vi "XY Graph Save Plot Event.vi"(6 "Delimiter (TAB)":string="\t", 8 "Error In":errorcluster, 9 "Mouse Click Coordinates":T1, 11 "XYGraph Ref":T2) -> (0 "Error Out":errorcluster, 1 "Message":string, 2 "File Path":path, 3 "Plot Name":string, 4 "Saved Plot Index":i32, 5 "Graph Caption":string)   [LabVIEW 2019, in "XY Graph Add-Ons.lvlib"]
uses:
  XY Graph Add-Ons.lvlib
  XY Graph Refnum.ctl
  <vilib>/Utility/miscctls.llb/LVPoint32TypeDef.ctl
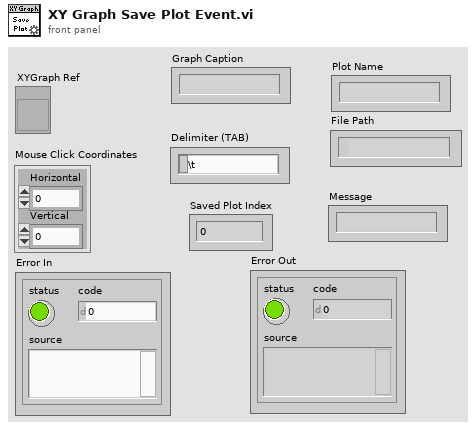
[diagram p1: front panel]
types:
  T1 = typedef "LVPoint32TypeDef.ctl" = cluster{"Horizontal":i32, "Vertical":i32}
  T2 = typedef "XY Graph Add-Ons.lvlib/XY Graph Refnum.ctl" = refnum<vi>
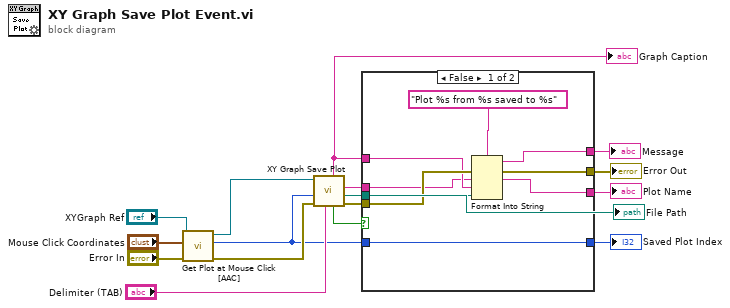
[diagram p0: block diagram]
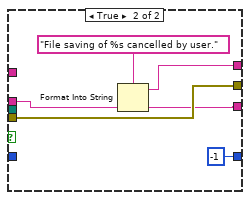
[diagram p2: hidden frame]
diagram:
  n1 = call "Get Plot at Mouse Click [AAC].vi"("error in (no error)"="Error In", "Mouse Click Coordinates"="Mouse Click Coordinates", "XYGraph Ref"="XYGraph Ref") -> ("error out"=w12:errorcluster, "Plot at Coordinates"=w3:i32, "XYGraph Ref"=w14:T2)  [unwired: 2 in, 4 out]
  n2 = call "XY Graph Save Plot.vi"("Delimiter (TAB)"="Delimiter (TAB)", "Error In"=w12, "Plot Index"=w3, "XYGraph Ref"=w14) -> ("Error Out"=w10:errorcluster, "File Path"=w9:path, "Plot Name"=w5:string, "Cancelled"=w4:bool, "Graph Name"=w6:string)  [unwired: 2 in, 1 out]
  "Graph Caption" <- w6
  "File Path" <- w9
  n3 = case shown="False" w4 {
    tunnel: w10 -> [w23 w29]
    tunnel: w9 -> [w22 _]
    tunnel: [w21 w29] -> w8
    tunnel: [w20 w25] -> w7
    tunnel: w6 -> [w19 _]
    tunnel: w5 -> [w17 w26]
    tunnel: w3 -> [w18 _]
    tunnel: [w18 -1 ("Plot at Coordinates")] -> w2
    tunnel: [w17 w26] -> w1
    frame False {
      n4 = Format Into String(format string="Plot %s from %s saved to %s", error in=w23, w17, w19, w22) -> (resulting string=w20:string, error out=w21:errorcluster)  [unwired: 1 in]
    }
    frame True {
      n5 = Format Into String(format string="File saving of %s cancelled by user.", w26) -> (resulting string=w25:string)  [unwired: 2 in, 1 out]
    }
  }
  "Error Out" <- w8
  "Saved Plot Index" <- w2
  "Plot Name" <- w1
  "Message" <- w7
